vi "2dArrayToFile.vi"(7 "advisory dialog? (display:T)":bool, 8 "Array":string[][](array[string]), 9 "file path (dialog if empty)":path) -> (3 "new file path (Not A Path if cancelled)":path)   [LabVIEW 2014, in "Panels.lvlib"]
uses:
  Panels.lvlib
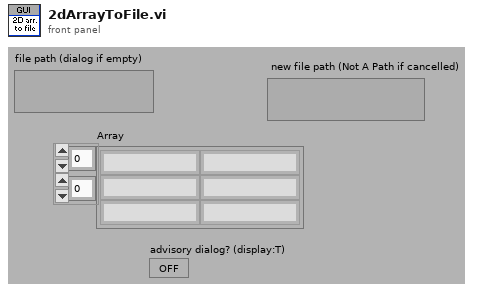
[diagram p1: front panel]
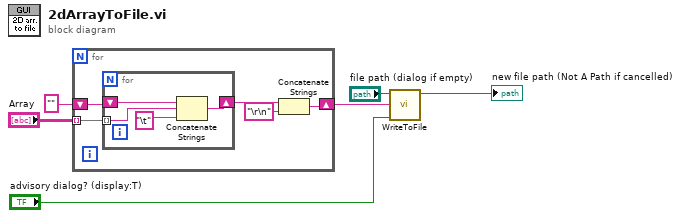
[diagram p0: block diagram]
diagram:
  n1 = for "For all Elements" {
    tunnel: "Array" -> [w11] mode=indexing
    shift-right: [w7] -> w4
    shift-left: "" -> [w10]
    n2 = for {
      tunnel: w11 -> [w14] mode=indexing
      shift-right: [w12] -> w9
      shift-left: w10 -> [w15]
      n3 = Concatenate Strings(w15, w14, "\t") -> (w12:string)
    }
    n4 = Concatenate Strings(w9, "\r\n") -> (w7:string)
  }
  n5 = call "WriteToFile.vi"("advisory dialog? (display:T)"="advisory dialog? (display:T)", "character string"=w4, "file path (dialog if empty)"="file path (dialog if empty)") -> ("new file path (Not A Path if cancelled)"=→"new file path (Not A Path if cancelled)":path)  [unwired: 7 in]
